vi "Waiting.vi"() -> ()   [LabVIEW 2020]
panel:
  out "Slide 2":cluster{u8, u8}(slide)={0, 47} scale=0.0..100.0
  in  "Numeric":u8
  out "Horizontal Progress Bar":cluster{u8, u8}(slide)={0, 32} scale=0.0..100.0
  in  "stop":bool
  out "Slide":cluster{u8, u8}(slide)={0, 47}
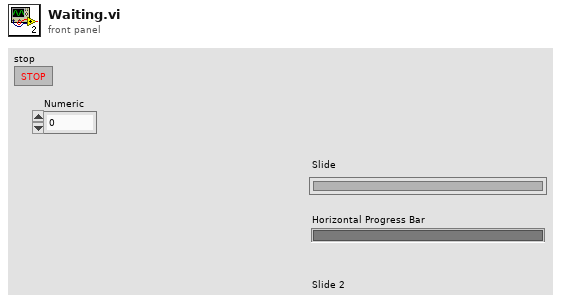
[diagram p1: front panel]
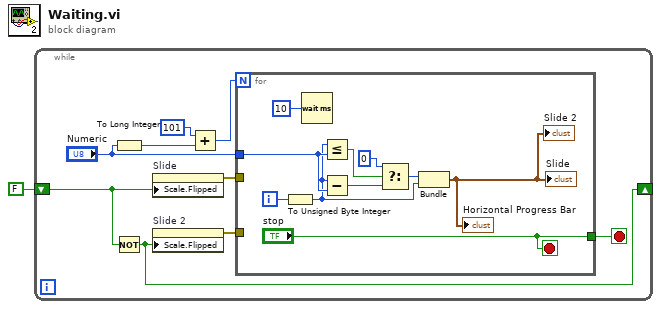
[diagram p0: block diagram]
diagram:
  n1 = while {
    shift-right: [w3] -> _
    shift-left: FALSE -> [w5]
    stop <- w10 stop-if-true
    n2 = To Long Integer(number="Numeric") -> (32bit integer=w6:i32)
    n3 = Not(x=w5) -> (.not. x?=w3:bool)
    n4 = property on="Slide" class="Slide (strict)"("Scale.Flipped"=w5) -> (error out=w4:errorcluster)  [unwired: 2 in, 1 out]
    n5 = property on="Slide 2" class="Slide (strict)"("Scale.Flipped"=w3) -> (error out=w2:errorcluster)  [unwired: 2 in, 1 out]
    n6 = Add(x=101, y=w6) -> (x+y=w8:i32)
    n7 = for {
      N: w8 -> [_]
      tunnel: ["stop"] -> w10
      tunnel: "Numeric" -> [w14]
      tunnel: w4 -> [_]
      tunnel: w2 -> [_]
      i -> [w15]
      stop <- "stop" stop-if-true
      n8 = To Unsigned Byte Integer(number=w15) -> (unsigned 8bit integer=w13:u8)
      n9 = Wait (ms)(milliseconds to wait=u32 10) -> ()  [unwired: 1 out]
      n10 = Less Or Equal?(x=w13, y=w14) -> (x <= y?=w16:bool)
      n11 = Subtract(x=w13, y=w14) -> (x-y=w19:u8)
      n12 = Select(t=u8 0, s=w16, f=w19) -> (s? t:f=w12:u8)
      n13 = Bundle("t"=w12, w13) -> (→"Slide" →"Horizontal Progress Bar" →"Slide 2":cluster{"t":u8, u8})  [unwired: 1 in]
    }
  }
